vi "Created.vi"(8 "Created Alias":string, 9 "Is Priority":bool, 10 "Msg":refnum<class "Msg.lvclass">, 11 "jettl Actor in":refnum<class "jettl Actor.lvclass">) -> (3 "jettl Actor out":refnum<class "jettl Actor.lvclass">)   [LabVIEW 2021, in "jettl.lvlib" / "Temporary Actor.lvlib" / "jettl Actor.lvclass"]
uses:
  jettl Actor.lvclass
  Msg/Msg.lvclass
  jettl Actor.lvclass/jettl Actor.ctl
  Utilities/Relation.ctl
  Addresses Strategy/Addresses Strategy/Addresses Strategy.lvclass
  Sender/Sender/Sender.lvclass
  Error/Error.lvlib
  Utilities/Utilities.lvlib
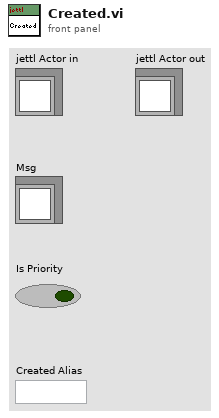
[diagram p1: front panel]
types:
  T1 = typedef "jettl.lvlib/Addresses Strategy.lvlib/Created.ctl" = map{string, refnum<user-event>}
  T2 = typedef "jettl.lvlib/Utilities.lvlib/Relation.ctl" = enum16{"Self", "Creator", "Created"}
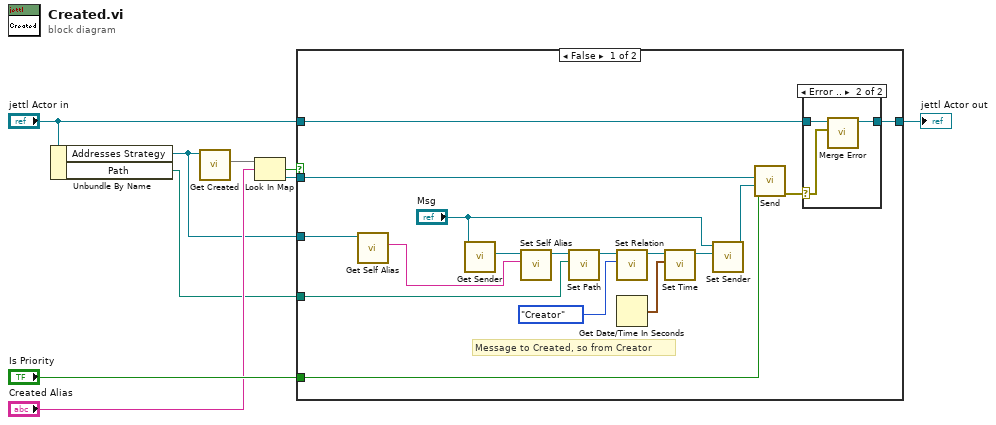
[diagram p0: block diagram]
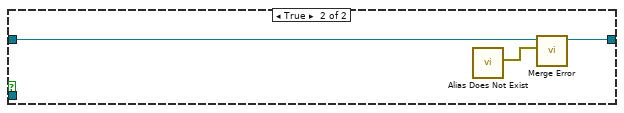
[diagram p3: hidden frame]
diagram:
  n1 = Unbundle By Name("jettl Actor in") -> ("Addresses Strategy"=w2:refnum<class "Addresses Strategy.lvclass">, "Path"=w1:path)
  n2 = call-dynamic "Get Created.vi"("Addresses Strategy in"=w2) -> ("Created"=w6:T1)  [unwired: 10 in]
  n3 = Look In Map(map=w6, key="Created Alias") -> (key not found?=w3:bool, value=w5:refnum<user-event>)  [unwired: 1 in]
  n4 = case shown="False" w3 {
    tunnel: "jettl Actor in" -> [w25 w33]
    tunnel: [w24 w32] -> w8
    tunnel: "Is Priority" -> [w23 _]
    tunnel: w5 -> [w22 _]
    tunnel: w2 -> [w20 _]
    tunnel: w1 -> [w11 _]
    frame False {
      # "Message to Created, so from Creator"
      n5 = call-dynamic "Get Self Alias.vi"("Addresses Strategy in"=w20) -> ("Self Alias"=w10:string)  [unwired: 10 in]
      n6 = call-dynamic "Get Sender.vi"("Msg in"="Msg") -> ("Sender"=w15:refnum<class "Sender.lvclass">)  [unwired: 10 in]
      n7 = call-dynamic "Set Self Alias.vi"("Self Alias"=w10, "Sender in"=w15) -> ("Sender out"=w16:refnum<class "Sender.lvclass">)  [unwired: 9 in]
      n8 = call-dynamic "Set Path.vi"("Path"=w11, "Sender in"=w16) -> ("Sender out"=w17:refnum<class "Sender.lvclass">)  [unwired: 9 in]
      n9 = call-dynamic "Set Relation.vi"("Relation"=Relation."Creator", "Sender in"=w17) -> ("Sender out"=w18:refnum<class "Sender.lvclass">)  [unwired: 9 in]
      n10 = Get Date/Time In Seconds() -> (seconds since 1Jan1904=w12:timestamp)
      n11 = call-dynamic "Set Time.vi"("Time"=w12, "Sender in"=w18) -> ("Sender out"=w14:refnum<class "Sender.lvclass">)  [unwired: 9 in]
      n12 = call-dynamic "Set Sender.vi"("Sender"=w14, "Msg in"="Msg") -> ("Msg out"=w21:refnum<class "Msg.lvclass">)  [unwired: 9 in]
      n13 = call "Send.vi"("Is Priority"=w23, "Msg"=w21, "Msg Event"=w22) -> ("error out"=w26:errorcluster)  [unwired: 8 in]
      n14 = case shown="Error .." w26 {
        selector: w26 -> [_ w28]
        tunnel: [w27 w30] -> w24
        tunnel: w25 -> [w27 w29]
        frame No Error {
        }
        frame Error {
          n15 = call-dynamic "Merge Error.vi"("Error"=w28, "jettl Actor in"=w29) -> ("jettl Actor out"=w30:refnum<class "jettl Actor.lvclass">)  [unwired: 9 in]
        }
      }
    }
    frame True {
      n16 = call "Alias Does Not Exist.vi"() -> ("Error"=w31:errorcluster)  [unwired: 11 in]
      n17 = call-dynamic "Merge Error.vi"("Error"=w31, "jettl Actor in"=w33) -> ("jettl Actor out"=w32:refnum<class "jettl Actor.lvclass">)  [unwired: 9 in]
    }
  }
  "jettl Actor out" <- w8
